vi "NI2564BOpenSession.vi"(8 "error in (no error)":errorcluster, 10 "gRPCid":T4, 11 "HVC9 In":T1) -> (0 "error out":errorcluster, 3 "HVC9 Out":T1)   [LabVIEW 2019, in "HVC9 User.lvlib"]
uses:
  HVC9 User.lvlib
  Servers/HVC9/gRPC lvSupport/Server API/typeDefs/grpcId.ctl
  Types/HVC9.ctl
  Types/HVC9 gRPC IDs.ctl
  Types/HVC9 Data.ctl
  Servers/HVC9/HVC9 Class/RPC Messages/measurementservice_NI2564OpenSessionResponse/measurementservice_NI2564OpenSessionResponse_Data.ctl
  Servers/HVC9/HVC9 Class/RPC Messages/measurementservice_ErrorOut/measurementservice_ErrorOut_Data.ctl
  Servers/HVC9/HVC9 Class/HVC9.lvclass
  Servers/HVC9/gRPC lvSupport/gprc-lvsupport.lvlib
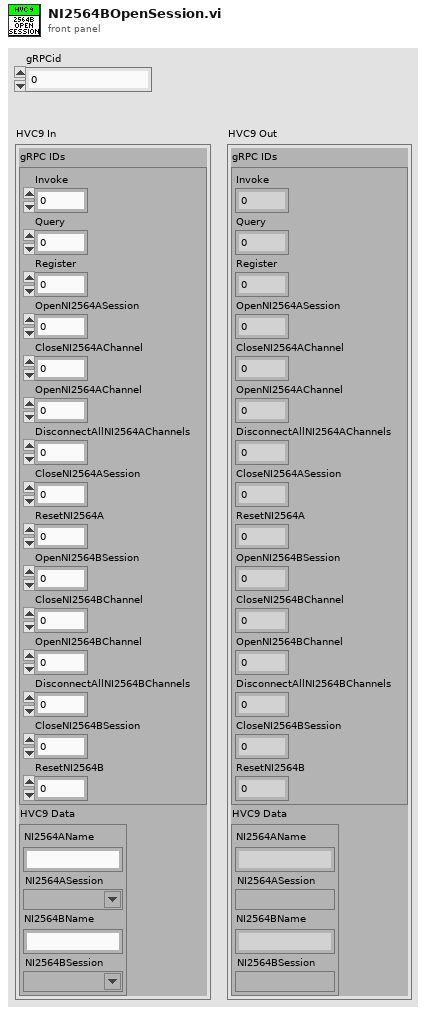
[diagram p1: front panel]
types:
  T1 = typedef "HVC9 User.lvlib/HVC9.ctl" = cluster{"gRPC IDs":T2, "HVC9 Data":T3}
  T2 = typedef "HVC9 User.lvlib/HVC9 gRPC IDs.ctl" = cluster{"Invoke ":u32, "Query":u32, "Register":u32, "OpenNI2564ASession":u32, "CloseNI2564AChannel ":u32, "OpenNI2564AChannel":u32, "DisconnectAllNI2564AChannels":u32, "CloseNI2564ASession":u32, "ResetNI2564A":u32, "OpenNI2564BSession":u32, "CloseNI2564BChannel ":u32, "OpenNI2564BChannel":u32, "DisconnectAllNI2564BChannels":u32, "CloseNI2564BSession":u32, "ResetNI2564B":u32}
  T3 = typedef "HVC9 User.lvlib/HVC9 Data.ctl" = cluster{"NI2564AName":string, "NI2564ASession":refnum<k15>, "NI2564BName":string, "NI2564BSession":refnum<k15>}
  T4 = typedef "HVC9.lvlib/gprc-lvsupport.lvlib/grpcId.ctl" = u64
  T5 = typedef "HVC9.lvlib/HVC9.lvclass/measurementservice_ErrorOut_Data.ctl" = cluster{"errCode":i32, "errMessage":string}
  T6 = typedef "HVC9.lvlib/HVC9.lvclass/measurementservice_NI2564OpenSessionResponse_Data.ctl" = cluster{"error":T5}
  T7 = typedef "HVC9.lvlib/HVC9.lvclass/measurementservice_NI2564OpenSessionRequest_Data.ctl" = cluster{"NI2564Name":string, "NI2564Topology":string}
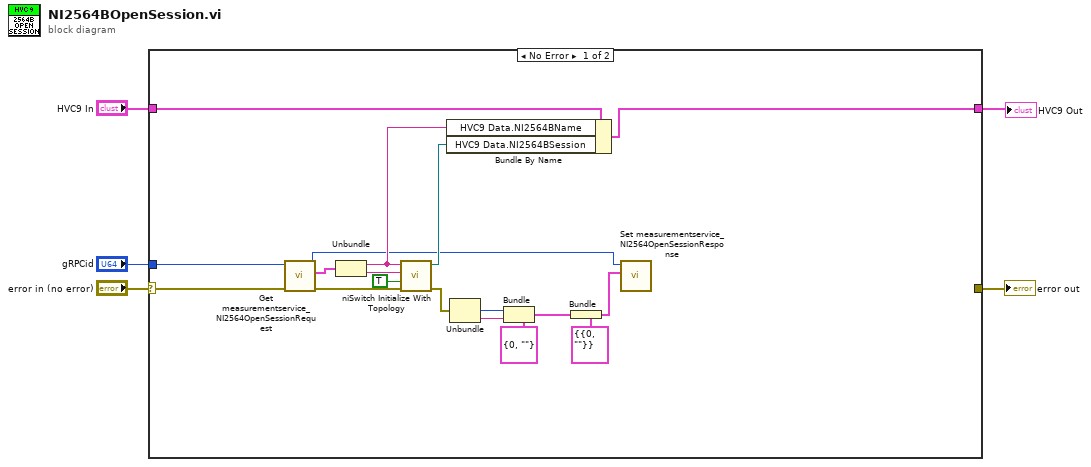
[diagram p0: block diagram]
diagram:
  n1 = case shown="No Error" "error in (no error)" {
    selector: "error in (no error)" -> [w8 w24]
    tunnel: [w22 w25] -> w1
    tunnel: "HVC9 In" -> [w20 w25]
    tunnel: "gRPCid" -> [w9 _]
    tunnel: [_ w24] -> w4
    frame No Error {
      n2 = call "Get measurementservice_NI2564OpenSessionRequest.vi"("error in (no error)"=w8, "gRPCid"=w9) -> ("error out"=w7:errorcluster, "Message Data"=w10:T7, "gRPCid out"=w11:T4)  [unwired: 7 in]
      n3 = Unbundle(w10) -> ("NI2564Name"=w23:string, "NI2564Topology"=w13:string)
      n4 = call <instrlib>:"niSwitch Initialize With Topology.vi"("error in (no error)"=w7, "reset device (boolean value)"=TRUE, "topology name"=w13, "resource name"=w23) -> ("error out"=w6:errorcluster, "instrument handle out"=w21:refnum<k15>)  [unwired: 6 in]
      n5 = Bundle By Name(cluster=w20, "HVC9 Data.NI2564BName"=w23, "HVC9 Data.NI2564BSession"=w21) -> (w22:T1)
      n6 = Unbundle(w6) -> ("code"=w16:i32, "source"=w17:string)  [unwired: 1 out]
      n7 = Bundle(cluster=T5 {"errCode"=0, "errMessage"=""} ("error"), "errCode"=w16, "errMessage"=w17) -> (w19:T5)
      n8 = Bundle(cluster=T6 {"error"={"errCode"=0, "errMessage"=""}} ("measurementservice_NI2564OpenSessionResponse_Data"), "error"=w19) -> (w15:T6)
      n9 = call "Set measurementservice_NI2564OpenSessionResponse.vi"("Message Data"=w15, "gRPCid"=w11) -> ()  [unwired: 9 in, 1 out]
    }
    frame Error {
    }
  }
  "error out" <- w4
  "HVC9 Out" <- w1
